vi "Subpanel.vi"() -> ()   [LabVIEW 2013]
uses:
  <vilib>/event_ctls.llb/eventvkey.ctl
  Global_Not-Aus.vi
panel:
  out "VKey":T1
  in  "Program Tab":enum32{"Page 1"}(tab)
  in  "Clear":bool
  in  "Stop Program":bool
  in  "Set Position":bool
  in  "Auto R/W":bool
  in  "Generate Script":bool
  in  "Read Sensors":bool
  out "Current Program":string
  in  "Title tab":enum32{"Page 1"}(tab)
  # "'Press' / click 'Esc' to stop\n           immediately"
  # "STOP"
  # "Write & Read Apparatus ( Control Panel )"
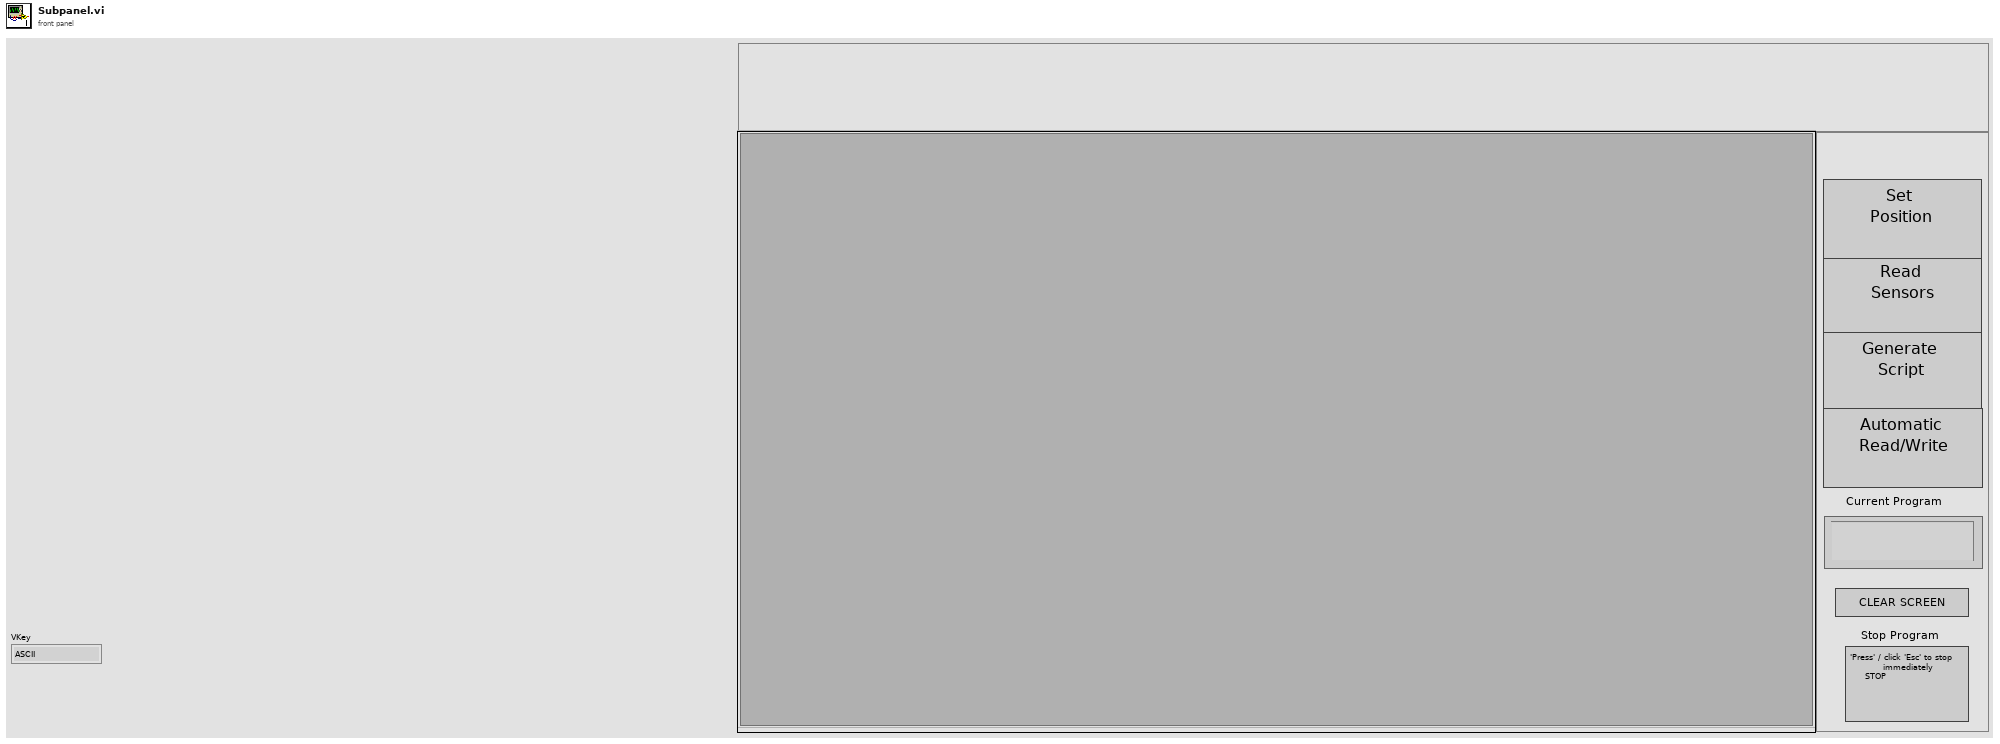
[diagram p1: front panel]
types:
  T1 = typedef "eventvkey.ctl" = enum16{"ASCII", "Enter", "Return", "Shift", "Ctrl", "Alt", "Cmd", "Opt", "Caps", "NumLock", "Clear", "Break", "Up", "Down", "Left", "Right", "Insert", "Delete", "Home", "End", "PageUp", "PageDown", "Escape", "Help", "Pause", "ScrollLock", "F1", "F2", "F3", "F4", "F5", "F6", "F7", "F8", "F9", "F10", "F11", "F12", "F13", "F14", "F15", "F16", "F17", "F18", "F19", "F20", "F21", "F22", "F23", "F24", "Play", "VolumeUp", "VolumeDown", "Mute", "Two Byte Char"}
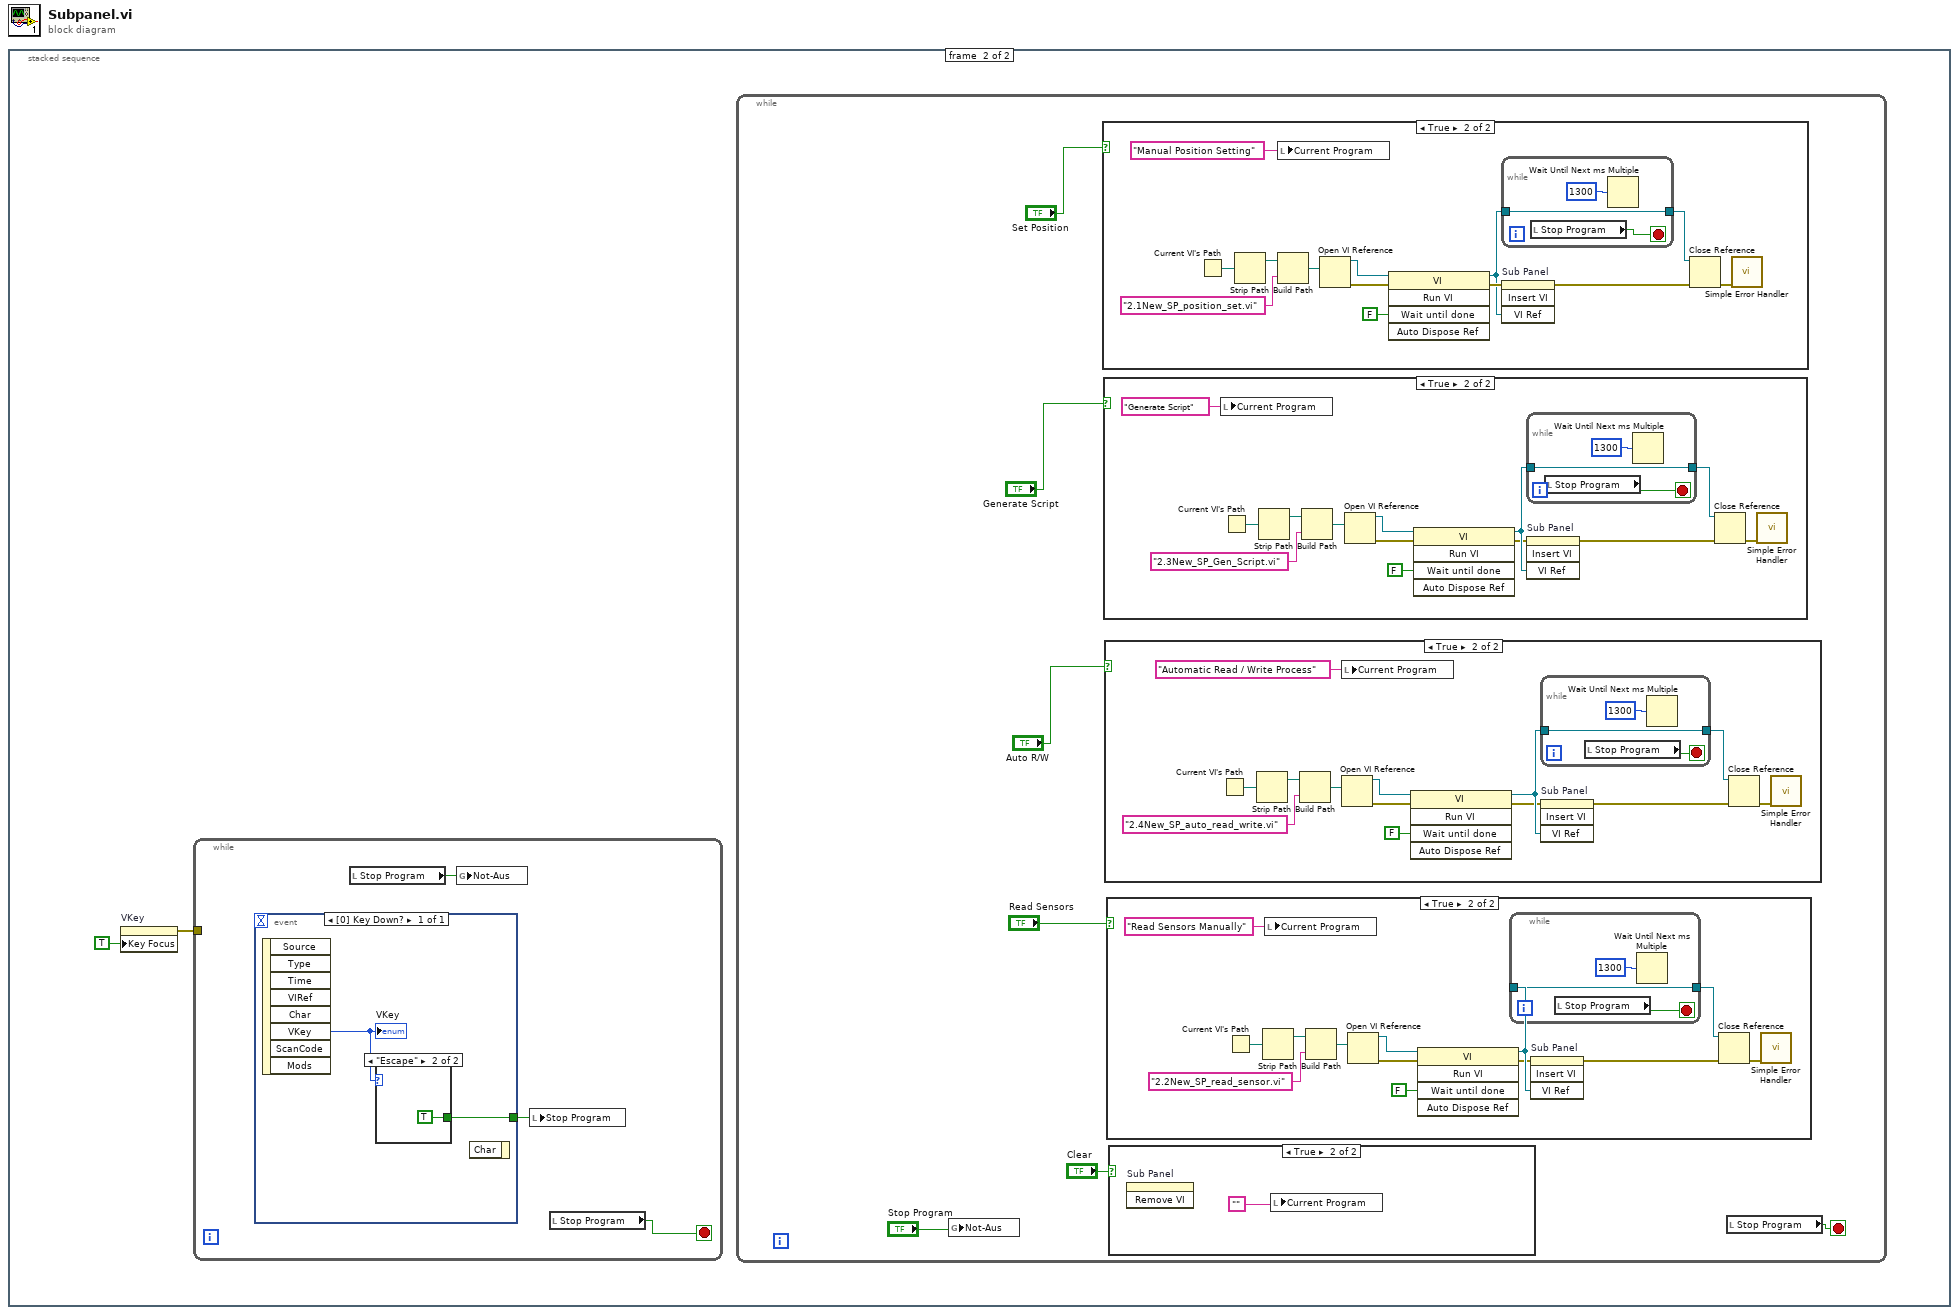
[diagram p0: block diagram]
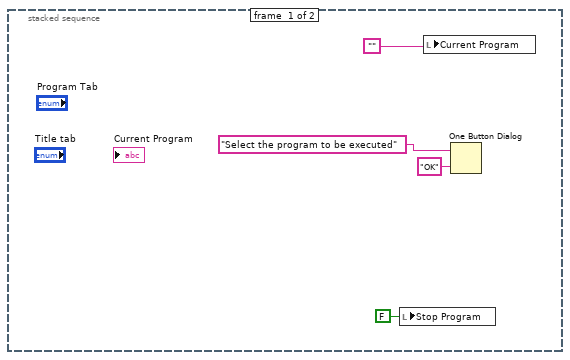
[diagram p2: hidden frame]
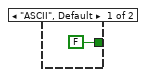
[diagram p3: hidden frame]
diagram:
  n1 = stacked-sequence {
    frame #0 {
      n2 = local write "Stop Program"(FALSE ("Stop Program")) -> ()
      n3 = local write "Current Program"("") -> ()
      n4 = One Button Dialog(message="Select the program to be executed" ("Current Program"), button name ("OK")="OK") -> ()  [unwired: 1 out]
    }
    frame #1 {
      n5 = property on="VKey" class="Enum (strict)"("Key Focus"=TRUE) -> (error out=w6:errorcluster)  [unwired: 2 in, 1 out]
      n6 = while {
        tunnel: w6 -> [_]
        stop <- w7 stop-if-true
        n7 = event shown="[0] Key Down?" {
          selector: _ -> [_]
          dyn-events: _ -> [_]
          timeout: _ -> [_]
          tunnel: [w11] -> w9
          event Key Down? {
            n8 = event-data() -> ("VKey"=w10:T1)  [unwired: 1 in, 7 out]
            "VKey" <- w10
            n9 = case shown="\"Escape\"" w10 {
              tunnel: [FALSE TRUE] -> w11
              frame "ASCII", Default {
              }
              frame "Escape" {
              }
            }
            n10 = event-data() -> ()  [unwired: 2 in, 1 out]
          }
        }
        n11 = local read "Stop Program"() -> (w8:bool)
        n12 = global write "Global_Not-Aus.vi" "Not-Aus"(w8) -> ()
        n13 = local write "Stop Program"(w9) -> ()
        n14 = local read "Stop Program"() -> (w7:bool)
      }
      n15 = while {
        stop <- w14 stop-if-true
        n16 = global write "Global_Not-Aus.vi" "Not-Aus"("Stop Program") -> ()
        n17 = case shown="True" "Set Position" {
          frame False {
          }
          frame True {
            n18 = Current VI's Path() -> (path=w76:path)
            n19 = Strip Path(path=w76) -> (stripped path=w75:path)  [unwired: 1 out]
            n20 = local write "Current Program"("Manual Position Setting" ("Current Program")) -> ()
            n21 = Build Path(base path=w75, name or relative path="2.1New_SP_position_set.vi") -> (appended path=w73:path)
            n22 = Open VI Reference(vi path=w73) -> (vi reference=w70:refnum<vi>, error out=w77:errorcluster)  [unwired: 5 in]
            n23 = invoke class="VI" method="Run VI"(reference=w70, error in=w77, "Wait until done"=FALSE ("Wait Until Done")) -> (reference out=w71:refnum<vi>, error out=w80:errorcluster)  [unwired: 2 in, 3 out]
            n24 = while {
              tunnel: [w84] -> w82
              tunnel: w71 -> [w84]
              stop <- w83 stop-if-true
              n25 = local read "Stop Program"() -> (w83:bool)
              n26 = Wait Until Next ms Multiple(millisecond multiple=u32 1300) -> ()  [unwired: 1 out]
            }
            n27 = invoke on="Sub Panel" class="SubPnl" method="Insert VI"(error in=w80, "VI Ref"=w71) -> (error out=w79:errorcluster)  [unwired: 2 in, 3 out]
            n28 = Close Reference(reference=w82, error in (no error)=w79) -> (error out=w78:errorcluster)
            n29 = call <vilib>:"Simple Error Handler.vi"("error in (no error)"=w78) -> ()  [unwired: 4 in, 5 out]
          }
        }
        n30 = case shown="True" "Generate Script" {
          frame False {
          }
          frame True {
            n31 = local write "Current Program"("Generate Script" ("Current Program")) -> ()
            n32 = Current VI's Path() -> (path=w58:path)
            n33 = Strip Path(path=w58) -> (stripped path=w57:path)  [unwired: 1 out]
            n34 = Build Path(base path=w57, name or relative path="2.3New_SP_Gen_Script.vi") -> (appended path=w55:path)
            n35 = Open VI Reference(vi path=w55) -> (vi reference=w65:refnum<vi>, error out=w59:errorcluster)  [unwired: 5 in]
            n36 = invoke class="VI" method="Run VI"(reference=w65, error in=w59, "Wait until done"=FALSE ("Wait Until Done")) -> (reference out=w63:refnum<vi>, error out=w61:errorcluster)  [unwired: 2 in, 3 out]
            n37 = while {
              tunnel: [w68] -> w66
              tunnel: w63 -> [w68]
              stop <- w67 stop-if-true
              n38 = local read "Stop Program"() -> (w67:bool)
              n39 = Wait Until Next ms Multiple(millisecond multiple=u32 1300) -> ()  [unwired: 1 out]
            }
            n40 = invoke on="Sub Panel" class="SubPnl" method="Insert VI"(error in=w61, "VI Ref"=w63) -> (error out=w60:errorcluster)  [unwired: 2 in, 3 out]
            n41 = Close Reference(reference=w66, error in (no error)=w60) -> (error out=w62:errorcluster)
            n42 = call <vilib>:"Simple Error Handler.vi"("error in (no error)"=w62) -> ()  [unwired: 4 in, 5 out]
          }
        }
        n43 = case shown="True" "Auto R/W" {
          frame False {
          }
          frame True {
            n44 = Current VI's Path() -> (path=w42:path)
            n45 = Strip Path(path=w42) -> (stripped path=w41:path)  [unwired: 1 out]
            n46 = Build Path(base path=w41, name or relative path="2.4New_SP_auto_read_write.vi") -> (appended path=w39:path)
            n47 = local write "Current Program"("Automatic Read / Write Process" ("Current Program")) -> ()
            n48 = Open VI Reference(vi path=w39) -> (vi reference=w49:refnum<vi>, error out=w43:errorcluster)  [unwired: 5 in]
            n49 = invoke class="VI" method="Run VI"(reference=w49, error in=w43, "Wait until done"=FALSE ("Wait Until Done")) -> (reference out=w47:refnum<vi>, error out=w45:errorcluster)  [unwired: 2 in, 3 out]
            n50 = while {
              tunnel: [w52] -> w50
              tunnel: w47 -> [w52]
              stop <- w51 stop-if-true
              n51 = local read "Stop Program"() -> (w51:bool)
              n52 = Wait Until Next ms Multiple(millisecond multiple=u32 1300) -> ()  [unwired: 1 out]
            }
            n53 = invoke on="Sub Panel" class="SubPnl" method="Insert VI"(error in=w45, "VI Ref"=w47) -> (error out=w44:errorcluster)  [unwired: 2 in, 3 out]
            n54 = Close Reference(reference=w50, error in (no error)=w44) -> (error out=w46:errorcluster)
            n55 = call <vilib>:"Simple Error Handler.vi"("error in (no error)"=w46) -> ()  [unwired: 4 in, 5 out]
          }
        }
        n56 = case shown="True" "Read Sensors" {
          frame False {
          }
          frame True {
            n57 = Current VI's Path() -> (path=w26:path)
            n58 = Strip Path(path=w26) -> (stripped path=w25:path)  [unwired: 1 out]
            n59 = local write "Current Program"("Read Sensors Manually" ("Current Program")) -> ()
            n60 = Build Path(base path=w25, name or relative path="2.2New_SP_read_sensor.vi") -> (appended path=w23:path)
            n61 = Open VI Reference(vi path=w23) -> (vi reference=w33:refnum<vi>, error out=w27:errorcluster)  [unwired: 5 in]
            n62 = invoke class="VI" method="Run VI"(reference=w33, error in=w27, "Wait until done"=FALSE ("Wait Until Done")) -> (reference out=w31:refnum<vi>, error out=w29:errorcluster)  [unwired: 2 in, 3 out]
            n63 = while {
              tunnel: [w36] -> w34
              tunnel: w31 -> [w36]
              stop <- w35 stop-if-true
              n64 = local read "Stop Program"() -> (w35:bool)
              n65 = Wait Until Next ms Multiple(millisecond multiple=u32 1300) -> ()  [unwired: 1 out]
            }
            n66 = invoke on="Sub Panel" class="SubPnl" method="Insert VI"(error in=w29, "VI Ref"=w31) -> (error out=w28:errorcluster)  [unwired: 2 in, 3 out]
            n67 = Close Reference(reference=w34, error in (no error)=w28) -> (error out=w30:errorcluster)
            n68 = call <vilib>:"Simple Error Handler.vi"("error in (no error)"=w30) -> ()  [unwired: 4 in, 5 out]
          }
        }
        n69 = case shown="True" "Clear" {
          frame False {
          }
          frame True {
            n70 = invoke on="Sub Panel" class="SubPnl" method="Remove VI"() -> ()  [unwired: 3 in, 3 out]
            n71 = local write "Current Program"("") -> ()
          }
        }
        n72 = local read "Stop Program"() -> (w14:bool)
      }
    }
  }
